vi "Read Attributes.vi"(0 "ILinked List in":refnum<class "ILinked List.lvclass">, 1 "Linked List ID":string, 3 "Include Private?":bool, 5 "Attribute Names":string[](array[string]), 9 "Flatten Pointer?":bool, 11 "error in (no error)":errorcluster) -> (4 "ILinked List out":refnum<class "ILinked List.lvclass">, 6 "Attribute Names out":string[](array[string]), 8 "Missing GUIDs out":string[](array[string]), 10 "Attributes":variant[](array[variant]), 12 "Found?":bool[](array[boolean]), 14 "Data IDs":string[](array[string]), 15 "error out":errorcluster)   [LabVIEW 2020, in "Linked Lists.lvlib" / "ILinked List.lvclass"]
uses:
  <vilib>/gpm_packages/@cs/linked-list/Source/Linked List/ILinkedList/ILinked List.lvclass
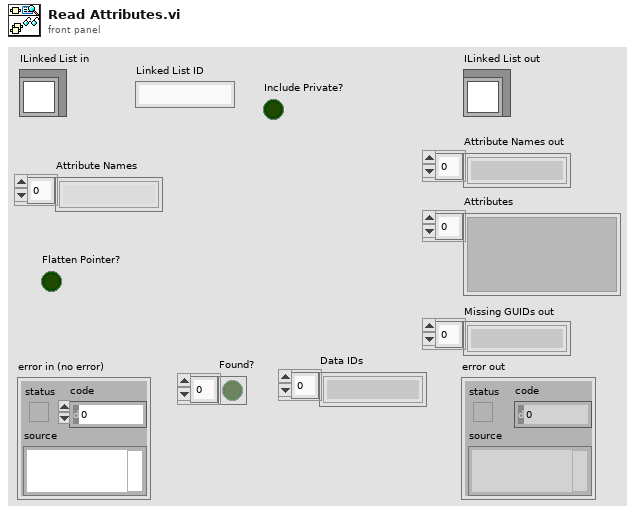
[diagram p1: front panel]
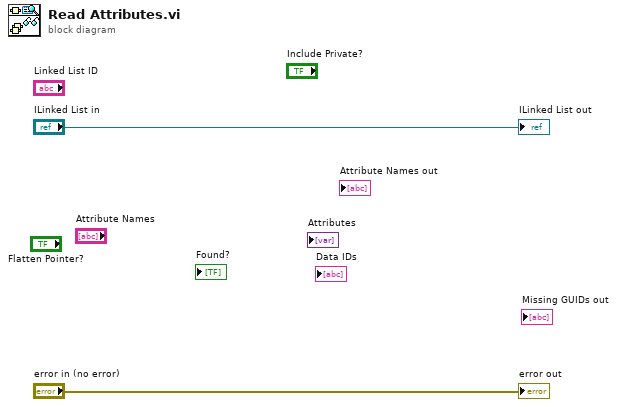
[diagram p0: block diagram]
diagram:
  "error out" <- "error in (no error)"
  "ILinked List out" <- "ILinked List in"
